vi "Get Spool Progress.vi"(11 "index":i32) -> (2 "function return":u32, 3 "index out":i32)   [LabVIEW 2018, in "AndorSDK.lvlib"]
doc: "EXPNETTYPE unsigned int WINAPI GetSpoolProgress(long * index);"
uses:
  AndorSDK.lvlib
  ATMCD32D.dll
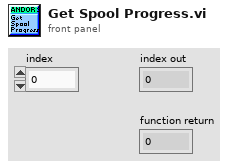
[diagram p1: front panel]
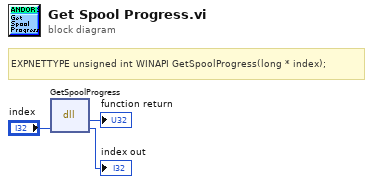
[diagram p0: block diagram]
diagram:
  # "EXPNETTYPE unsigned int WINAPI GetSpoolProgress(long * index);"
  n1 = dll-call lib="PTH2babs E\nPersönliches02 - Arbeit03-HiwijobsLabviewCodelibANDOR\tAndor SDK\nATMCD32D.*" fn="GetSpoolProgress"("index"="index") -> (→"function return":u32, "index"=→"index out":i32)  [unwired: 3 in, 2 out]
